vi "draw rectangles.vi"(3 "Image":T2, 4 "error in (no error)":errorcluster, 5 "Array":i32[][](array[numeric])) -> (0 "error out":errorcluster, 1 "Image Pixels (U8)":u8[][](array[numeric]))   [LabVIEW 2011]
uses:
  <vilib>/vision/Image Controls.llb/IMAQ Image.ctl
  <vilib>/vision/NI_Vision_Development_Module.lvlib
panel:
  in  "Font, Size & Style":T1={"Desired Font (Application)"=enum."User-specified Font", "[User-specified Font]"={"Font Name"="Times", "Size"=30, "Strikeout?"=FALSE, "Italic?"=FALSE, "Underline?"=FALSE, "Outline?"=FALSE, "Shadow?"=FALSE, "Bold?"=FALSE, "Rotation Angle"=0.0}, "Horizontal Alignment"=0, "Vertical Alignment"=0} {"Horizontal Alignment" items=["Left", "Center", "Right"]; "Vertical Alignment" items=["Bottom", "Top", "Baseline"]}
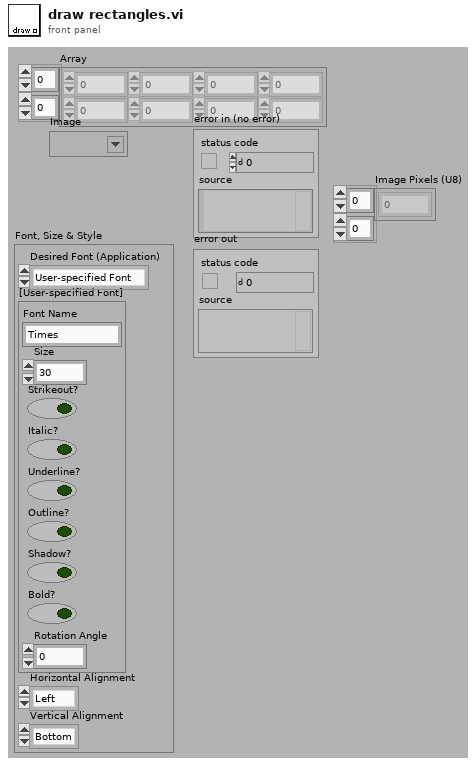
[diagram p1: front panel]
types:
  T1 = cluster{"Desired Font (Application)":enum16{"User-specified Font", "Application Font", "System Font", "Dialog Font"}, "[User-specified Font]":cluster{"Font Name":string, "Size":i16, "Strikeout?":bool, "Italic?":bool, "Underline?":bool, "Outline?":bool, "Shadow?":bool, "Bold?":bool, "Rotation Angle":dbl}, "Horizontal Alignment":i16, "Vertical Alignment":i16}
  T2 = typedef "IMAQ Image.ctl" = refnum<image>
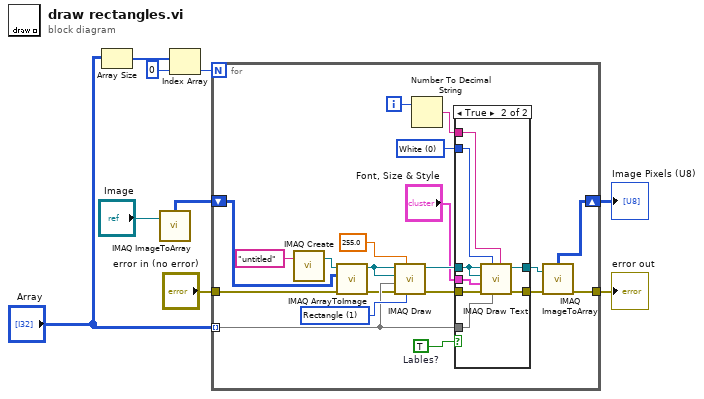
[diagram p0: block diagram]
diagram:
  n1 = Array Size(array="Array") -> (size(s)=w7:i32[])
  n2 = call "IMAQ ImageToArray"("Image"="Image") -> ("Image Pixels (U8)"=w3:u8[][])  [unwired: 2 in, 5 out]
  n3 = Index Array(array=w7, index=0) -> (element=w6:i32)
  n4 = for {
    N: w6 -> [_]
    tunnel: "Array" -> [w19] mode=indexing
    shift-right: [w25] -> w9
    shift-left: w3 -> [w29]
    tunnel: "error in (no error)" -> [w16]
    tunnel: [w12] -> w1
    i -> [w22]
    w10 = TRUE  # Lables?
    w20 = 0 items=["White", "Black", "Inverted", "Black on White", "White on Black"] ("Color")
    w27 = u16 1 items=["Line", "Rectangle", "Oval"] ("Shape to draw")
    n5 = call "IMAQ Create"("Image Name"="untitled") -> ("New Image"=w18:T2)  [unwired: 3 in, 2 out]
    n6 = call "IMAQ ArrayToImage"("error in (no error)"=w16, "Image Pixels (U8)"=w29, "Image"=w18) -> ("error out"=w15:errorcluster, "Image Out"=w28:T2)  [unwired: 3 in, 4 out]
    n7 = call "IMAQ Draw"("Shape to draw"=w27, "Pixel Color"=sgl 255.0, "error in (no error)"=w15, "Coordinates"=w19, "Image Dst"=w28, "Image Src"=w28) -> ("error out"=w14:errorcluster, "Image Dst Out"=w24:T2)  [unwired: 1 in, 3 out]
    n8 = Number To Decimal String(number=w22) -> (decimal integer string=w21:string)  [unwired: 1 out]
    n9 = case shown="True" w10 {
      tunnel: w24 -> [w31 w39]
      tunnel: [w31 w38] -> w23
      tunnel: w21 -> [_ w37]
      tunnel: w20 -> [_ w36]
      tunnel: w19 -> [_ w35]
      tunnel: w14 -> [w30 w34]
      tunnel: [w30 w33] -> w13
      tunnel: "Font, Size & Style" -> [_ w32]
      frame False {
      }
      frame True {
        n10 = call "IMAQ Draw Text"("String"=w37, "Insertion Point"=w35, "Color"=w36, "error in (no error)"=w34, "Font, Size & Style"=w32, "Image Dst"=w39, "Image Src"=w39) -> ("error out"=w33:errorcluster, "Image Dst Out"=w38:T2)  [unwired: 3 out]
      }
    }
    n11 = call "IMAQ ImageToArray"("error in (no error)"=w13, "Image"=w23) -> ("error out"=w12:errorcluster, "Image Pixels (U8)"=w25:u8[][])  [unwired: 1 in, 4 out]
  }
  "Image Pixels (U8)" <- w9
  "error out" <- w1
